vi "Set state (subVi).vi"() -> ()   [LabVIEW 2016]
uses:
  global/Config_Infos.vi
panel:
  out "path":path
  out "element":string
  in  "Array - String":string[](array[string])=["FilOff_SavingOff", "FilOn_SavingOff", "FilOn_SavingOn"]
  out "error out":errorcluster
  in  "source path":path
  in  "path (use dialog)":path
  in  "Text Ring":u16(ring) items=["Filament off/Saving off", "Filament on/Saving off", "Filament on/Saving on"]
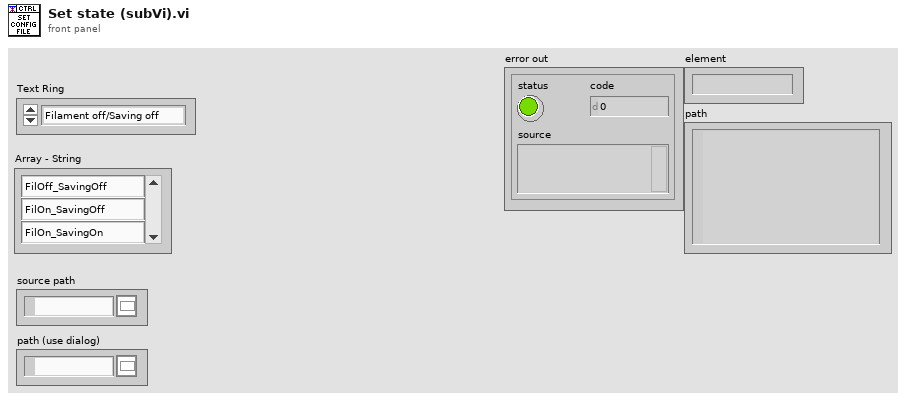
[diagram p1: front panel]
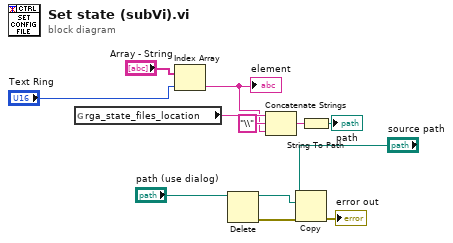
[diagram p0: block diagram]
diagram:
  n1 = global read "Config_Infos.vi" "rga_state_files_location"() -> (w5:string)
  n2 = Index Array(array="Array - String", index="Text Ring") -> (element=w3:string)
  "element" <- w3
  n3 = Delete(path (use dialog)="path (use dialog)") -> (deleted path=w11:path, error out=w9:errorcluster)  [unwired: 4 in, 1 out]
  n4 = Concatenate Strings(w5, "\\" ("string"), w3) -> (w2:string)
  n5 = Copy(8:w9, 10:w11, 11:"source path") -> (0:→"error out":errorcluster)  [unwired: 2 in, 2 out]
  n6 = String To Path(string=w2) -> (path=→"path":path)
